vi "Flatten SubVI.vi"(4 "Condensed?":bool, 6 "No Label?":bool, 8 "error in (no error)":errorcluster, 11 "Data":variant) -> (0 "error out":errorcluster, 3 "YAML String out":string)   [LabVIEW 2015, in "YAML Parser.lvclass"]
uses:
  YAML Parser.lvclass
  <vilib>/Utility/Data Type/NI_Data Type.lvlib
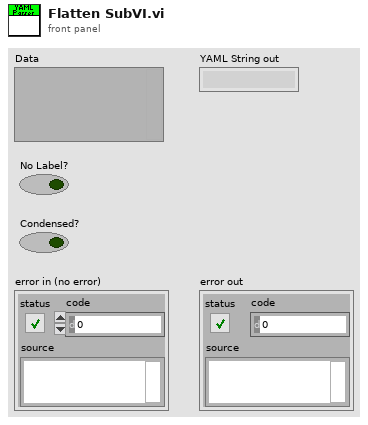
[diagram p1: front panel]
types:
  T1 = typedef "NI_Data Type.lvlib/Data Type.ctl" = enum8{"Invalid Type", "Void", "I8", "I16", "I32", "I64", "U8", "U16", "U32", "U64", "Single Float", "Double Float", "Extended Float", "Single Complex", "Double Complex", "Extended Complex", "Enum U8", "Enum U16", "Enum U32", "Enum U64", "Single Float With Unit", "Double Float With Unit", "Extended Float With Unit", "Single Complex with Unit", "Double Complex with Unit", "Extended Complex with Unit", "Boolean", "String", "Path", "Picture", "Tag", "Array", "Cluster", "Variant", "LV Variant", "Waveform", "Timestamp", "Digital Waveform", "Digital Data", "ExpressData", "Refnum", "External Data", "VI", "Poly VI", "LabVIEW Class Instance", "Fixed Point"}
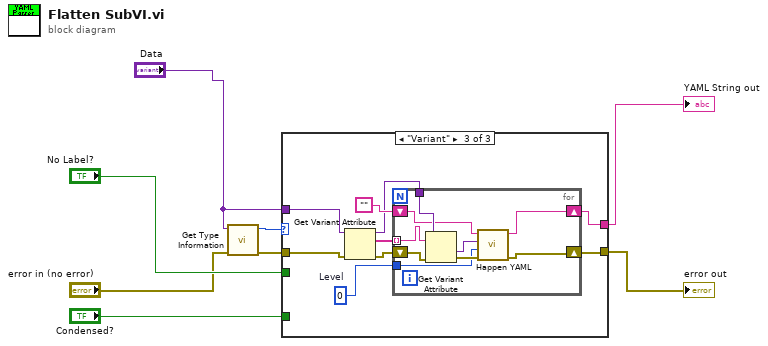
[diagram p0: block diagram]
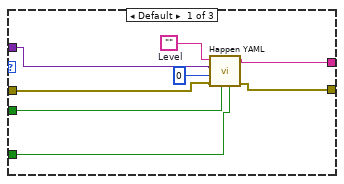
[diagram p2: hidden frame]
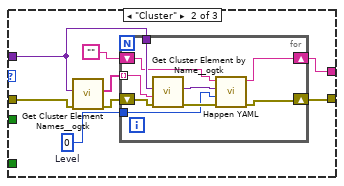
[diagram p3: hidden frame]
diagram:
  n1 = call <vilib>:"Get Type Information.vi"("error in (no error)"="error in (no error)", "Variant"="Data") -> ("error out"=w8:errorcluster, "Type"=w7:T1)  [unwired: 5 in, 3 out]
  n2 = case shown="\"Variant\"" w7 {
    tunnel: w8 -> [w11 w20 w38]
    tunnel: "Data" -> [w14 w17 w37]
    tunnel: [w16 w24 w42] -> w2
    tunnel: [w15 w23 w41] -> w4
    tunnel: "No Label?" -> [w10 _ _]
    tunnel: "Condensed?" -> [w9 _ _]
    frame Default {
      w13 = u32 0  # Level
      n3 = call "Happen YAML.vi"("Condensed?"=w9, "No Label?"=w10, "error in (no error)"=w11, "Level"=w13, "Anything"=w14, "YAML String in"="") -> ("error out"=w16:errorcluster, "YAML String out"=w15:string)  [unwired: 4 in]
    }
    frame "Cluster" {
      w21 = u32 0  # Level
      n4 = call <userlib>:"Get Cluster Element Names__ogtk.vi"("error in (no error)"=w20, "Cluster"=w17) -> ("error out"=w19:errorcluster, "Element Names"=w18:string[])  [unwired: 8 in]
      n5 = for {
        tunnel: w18 -> [w31] mode=indexing
        shift-right: [w30] -> w24
        shift-left: w19 -> [w33]
        shift-right: [w29] -> w23
        shift-left: "" -> [w28]
        tunnel: w21 -> [w26]
        tunnel: w17 -> [w32]
        n6 = call <userlib>:"Get Cluster Element by Name__ogtk.vi"("error in (no error)"=w33, "Element Name"=w31, "Cluster"=w32) -> ("error out"=w27:errorcluster, "VElement"=w25:variant)  [unwired: 6 in, 1 out]
        n7 = call "Happen YAML.vi"("error in (no error)"=w27, "Level"=w26, "Anything"=w25, "YAML String in"=w28) -> ("error out"=w30:errorcluster, "YAML String out"=w29:string)  [unwired: 6 in]
      }
    }
    frame "Variant" {
      w39 = u32 0  # Level
      n8 = Get Variant Attribute(Variant=w37, error in=w38) -> (duplicate Variant=w36:variant, names=w34:string[], error out=w35:errorcluster)  [unwired: 2 in, 1 out]
      n9 = for {
        shift-right: [w48] -> w42
        shift-left: w35 -> [w51]
        shift-right: [w43] -> w41
        shift-left: "" -> [w44]
        tunnel: w39 -> [w45]
        tunnel: w36 -> [w49]
        tunnel: w34 -> [w50] mode=indexing
        n10 = Get Variant Attribute(Variant=w49, name=w50, error in=w51) -> (value=w46:variant, error out=w47:errorcluster)  [unwired: 1 in, 2 out]
        n11 = call "Happen YAML.vi"("error in (no error)"=w47, "Level"=w45, "Anything"=w46, "YAML String in"=w44) -> ("error out"=w48:errorcluster, "YAML String out"=w43:string)  [unwired: 6 in]
      }
    }
  }
  "YAML String out" <- w4
  "error out" <- w2
